vi "Get Boards List.vi"(8 "error in (no error)":errorcluster, 11 "Platform in":refnum<class "DeployPlatform.lvclass">) -> (0 "error out":errorcluster, 2 "Boards":string[](array[string]), 3 "Platform out":refnum<class "DeployPlatform.lvclass">)   [LabVIEW 2020, in "PicoG-Core.lvlib" / "DeployPlatform.lvclass"]
uses:
  DeployPlatform.lvclass
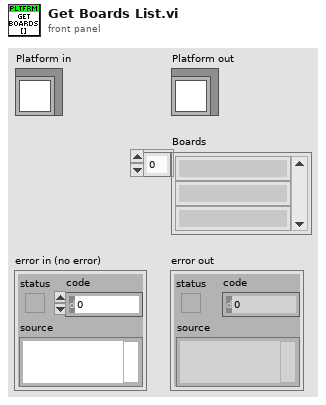
[diagram p1: front panel]
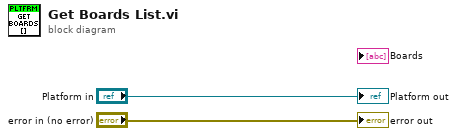
[diagram p0: block diagram]
diagram:
  "error out" <- "error in (no error)"
  "Platform out" <- "Platform in"
